vi "sv_UFF58 Init Function.vi"(0 "file refnum":refnum<k20>, 11 "error in (no error)":errorcluster) -> (4 "dup file refnum":refnum<k20>, 6 "function refnum":refnum<k20>, 15 "error out":errorcluster)   [LabVIEW 2017, in "SoundVib_UFF58.lvlib"]
doc: "This function create a <B>function refnum</B> for the given <B>file refnum</B>"
uses:
  <vilib>/addons/Sound and Vibration/svt_UFF58/SoundVib_UFF58.lvlib
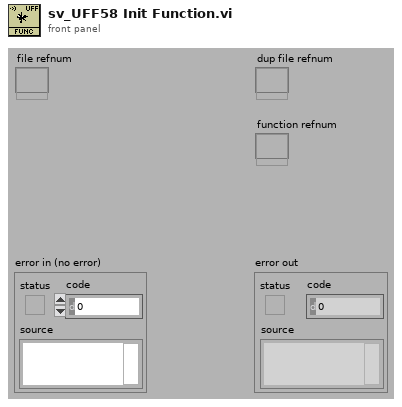
[diagram p1: front panel]
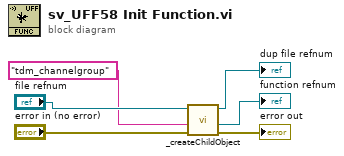
[diagram p0: block diagram]
diagram:
  n1 = call <vilib>:"_createChildObject.vi"("error in (no error)"="error in (no error)", "Object type"="tdm_channelgroup", "storage refnum"="file refnum") -> ("error out"=→"error out":errorcluster, "new storage refnum"=→"function refnum":refnum<k20>, "dup storage refnum"=→"dup file refnum":refnum<k20>)  [unwired: 2 in]
